vi "getObject.vi"(0 "reference":refnum<class "Direction.lvclass">, 1 "direction":T1, 5 "error in (no error)":errorcluster) -> (14 "reference out":refnum<class "Direction.lvclass">, 15 "directionRef":refnum<class "Direction.lvclass">, 19 "error out":errorcluster)   [LabVIEW 2012, in "Direction.lvclass"]
doc: "Gets an Object"
uses:
  <resource>/Framework/Providers/Open_GDS/UML/Direction_class/Direction.lvclass
  <resource>/Framework/Providers/Open_GDS/UML/Direction_class/DirectionTypes.ctl
  <resource>/Framework/Providers/Open_GDS/UML/General/Point/Point Point2D.ctl
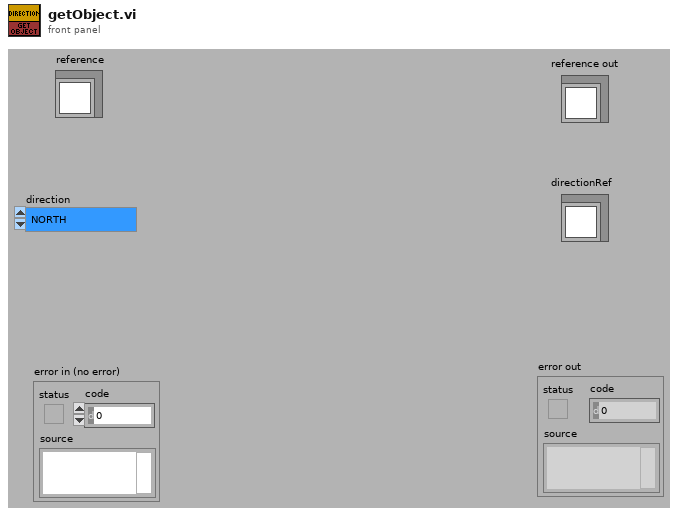
[diagram p1: front panel]
types:
  T1 = typedef "Direction.lvclass/DirectionTypes.ctl" = enum16{"NORTH", "SOUTH", "EAST", "WEST"}
  T2 = typedef "Point Point2D.ctl" = cluster{"x":dbl, "y":dbl}
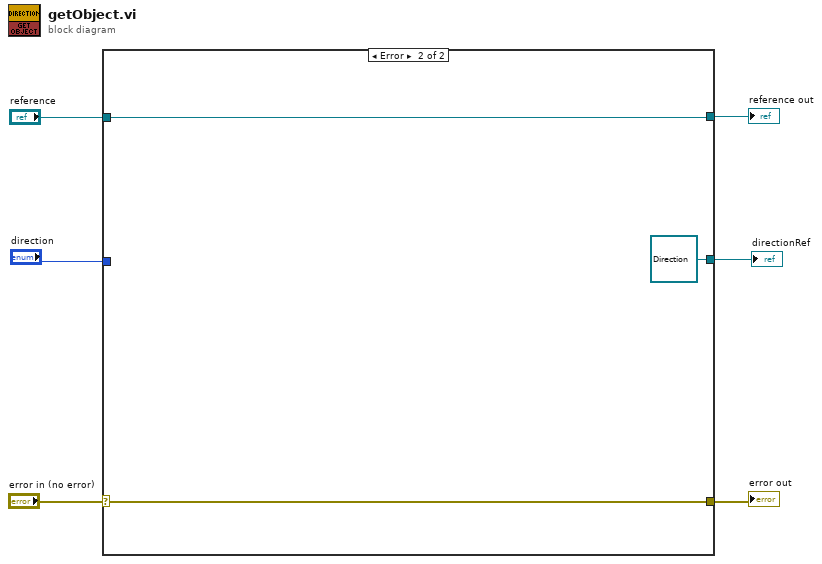
[diagram p0: block diagram]
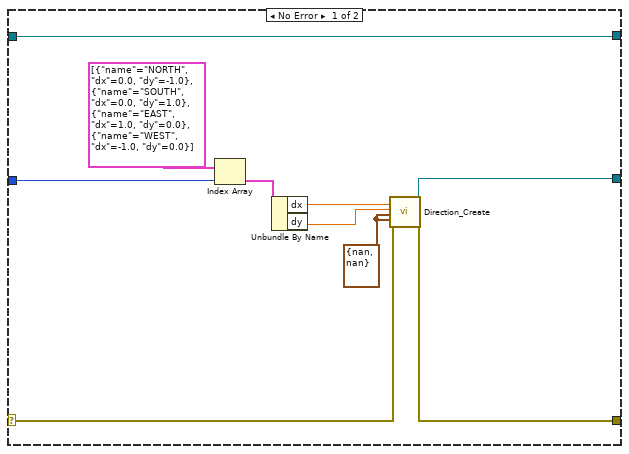
[diagram p2: hidden frame]
diagram:
  n1 = case shown="Error" "error in (no error)" {
    selector: "error in (no error)" -> [w15 w18]
    tunnel: "reference" -> [w16 w19]
    tunnel: [w14 w18] -> w4
    tunnel: [w16 w19] -> w3
    tunnel: [w8 refnum<class "Direction.lvclass"> refnum ("reference out")] -> w2
    tunnel: "direction" -> [w13 _]
    frame No Error {
      w7 = T2 {"x"=nan, "y"=nan} ("p1")
      n2 = Index Array(array=cluster{"name":string, "dx":dbl, "dy":dbl}[] [{"name"="NORTH", "dx"=0.0, "dy"=-1.0}, {"name"="SOUTH", "dx"=0.0, "dy"=1.0}, {"name"="EAST", "dx"=1.0, "dy"=0.0}, {"name"="WEST", "dx"=-1.0, "dy"=0.0}], index=w13) -> (element=w11:cluster{"name":string, "dx":dbl, "dy":dbl})
      n3 = Unbundle By Name(w11) -> ("dx"=w10:dbl, "dy"=w9:dbl)
      n4 = call <resource>:"Direction_Create.vi"("dx"=w10, "dy"=w9, "p1"=w7, "p2"=w7, "error in (no error)"=w15) -> ("reference out"=w8:refnum<class "Direction.lvclass">, "error out"=w14:errorcluster)  [unwired: 13 in]
    }
    frame Error {
    }
  }
  "reference out" <- w3
  "error out" <- w4
  "directionRef" <- w2
